vi "Run ProviderVI.vi"(7 "Shell VI":refnum<vi>, 8 "error in (no error)":errorcluster, 11 "vi reference":refnum<vi>) -> (0 "error out":errorcluster, 3 "VI out":refnum<vi>)   [LabVIEW 2019, in "LabVIEW-ProviderShell.lvlib" / "LvProviderShellHelper.lvclass"]
uses:
  LvProviderShellHelper.lvclass
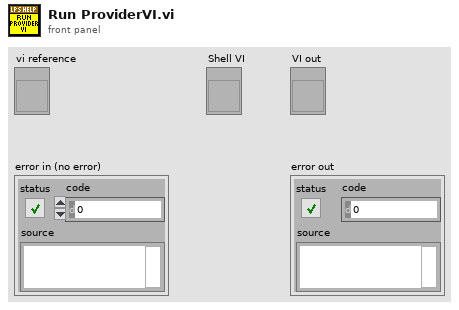
[diagram p1: front panel]
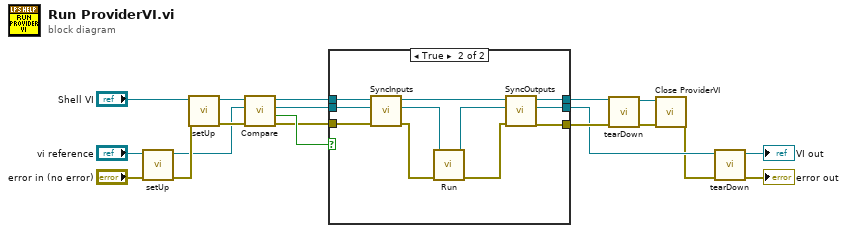
[diagram p0: block diagram]
diagram:
  n1 = call "setUp.vi"("error in (no error)"="error in (no error)", "VI in"="vi reference") -> ("error out"=w9:errorcluster, "fpMgr out"=w2:refnum<class "LvProviderShellHelper.lvclass">)  [unwired: 8 in]
  n2 = call "setUp.vi"("error in (no error)"=w9, "VI in"="Shell VI") -> ("error out"=w3:errorcluster, "fpMgr out"=w1:refnum<class "LvProviderShellHelper.lvclass">)  [unwired: 8 in]
  n3 = call "Compare.vi"("error in (no error)"=w3, "fpMgr in"=w2, "Shell in"=w1) -> ("error out"=w15:errorcluster, "Matched"=w19:bool, "fpMgr out"=w12:refnum<class "LvProviderShellHelper.lvclass">, "Shell out"=w10:refnum<class "LvProviderShellHelper.lvclass">)  [unwired: 5 in]
  n4 = case shown="True" w19 {
    tunnel: w10 -> [w22 w33]
    tunnel: [w22 w31] -> w11
    tunnel: w12 -> [w20 w30]
    tunnel: [w20 w27] -> w13
    tunnel: [w21 w26] -> w14
    tunnel: w15 -> [w21 w25]
    frame False {
    }
    frame True {
      n5 = call "SyncInputs.vi"("error in (no error)"=w25, "fpMgr in"=w30, "Shell in"=w33) -> ("error out"=w24:errorcluster, "fpMgr out"=w29:refnum<class "LvProviderShellHelper.lvclass">, "Shell out"=w32:refnum<class "LvProviderShellHelper.lvclass">)  [unwired: 6 in]
      n6 = call "Run.vi"("error in (no error)"=w24, "fpMgr in"=w29) -> ("error out"=w23:errorcluster, "fpMgr out"=w28:refnum<class "LvProviderShellHelper.lvclass">)  [unwired: 8 in]
      n7 = call "SyncOutputs.vi"("error in (no error)"=w23, "fpMgr in"=w28, "Shell in"=w32) -> ("error out"=w26:errorcluster, "fpMgr out"=w27:refnum<class "LvProviderShellHelper.lvclass">, "Shell out"=w31:refnum<class "LvProviderShellHelper.lvclass">)  [unwired: 6 in]
    }
  }
  n8 = call "tearDown.vi"("error in (no error)"=w14, "fpMgr in"=w11) -> ("error out"=w5:errorcluster, "VI"=w4:refnum<vi>)  [unwired: 8 in]
  n9 = call "Close ProviderVI.vi"("error in (no error)"=w5, "VI in"=w4) -> ("error out"=w6:errorcluster)  [unwired: 9 in]
  n10 = call "tearDown.vi"("error in (no error)"=w6, "fpMgr in"=w13) -> ("error out"=→"error out":errorcluster, "VI"=→"VI out":refnum<vi>)  [unwired: 8 in]
